vi "Arduino_Serial_GlobalConstants.vi"() -> ()   [LabVIEW 2012]
panel:
  in  "Packet Number":u16=1
  in  "Length of Command Field":i32=4
  in  "NACK Number":i32=21
  in  "ACK Number":i32=6
  in  "Protocol Version":string="01"
  in  "NACK Char":string="\u0015"
  in  "ACK Char":string="\u0006"
  in  "ETX Char":string="\u0003"
  in  "STX Char":string="\u0002"
  in  "Length of End Field":i32=1
  in  "Length of CRC Field":i32=4
  in  "Length of PacketNum Field":i32=4
  in  "Length of Control Field":i32=2
  in  "Length of Protocol Revision":i32=2
  in  "Length of Length Field":i32=4
  in  "Length of STX field":i32=1
  # "CONSTANTS FOR SERIAL PROTOCOL"
  # "VARIABLES FOR SERIAL PROTOCOL DURING OPERATION"
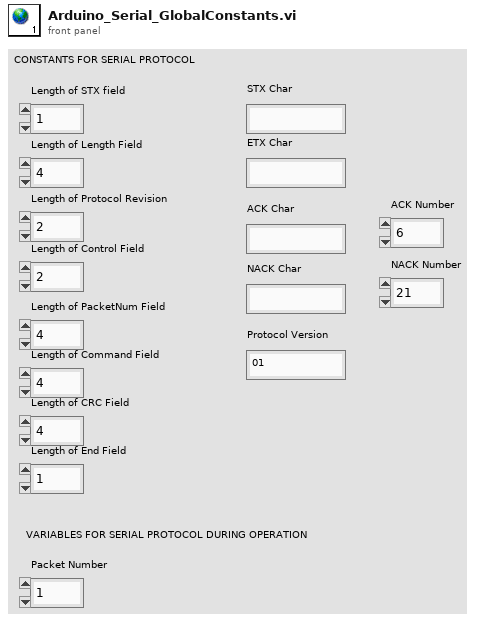
[diagram p1: front panel]
diagram:
